vi "testCQTDDSlabview.vi"() -> ()   [LabVIEW 2009, in "run.lvlib"]
uses:
  run.lvlib
  Channels/DDSOutput/Generic/DDSOutput.lvclass
panel:
  in  "Phase 2":dbl[](array[numeric])=[0.0, 0.0, 0.0]
  in  "Amp 2":dbl[](array[numeric])=[1.0, 1.0, 0.0]
  in  "freq 2":dbl[](array[numeric])=[100.0, 90.0, 100.0]
  in  "Phase":dbl[](array[numeric])=[0.0, 0.0, 0.0]
  in  "Amp":dbl[](array[numeric])=[1.0, 1.0, 0.0]
  in  "freq":dbl[](array[numeric])=[100.0, 90.0, 100.0]
  in  "Times":dbl[](array[numeric])=[0.0, 1.0, 2.0]
  in  "stop":bool
  in  "physicalChannels":string[](array[string])=["CQTDDS0_rf_00", "CQTDDS0_rf_01"]
  in  "data":T1(array[cluster])=[{"Frequency(MHz)"=10.0, "Amplitude"=1.0, "Phase"=0.0, "OutputForm"=enum."Sine"}, {"Frequency(MHz)"=10.0, "Amplitude"=1.0, "Phase"=180.0, "OutputForm"=enum."Sine"}]
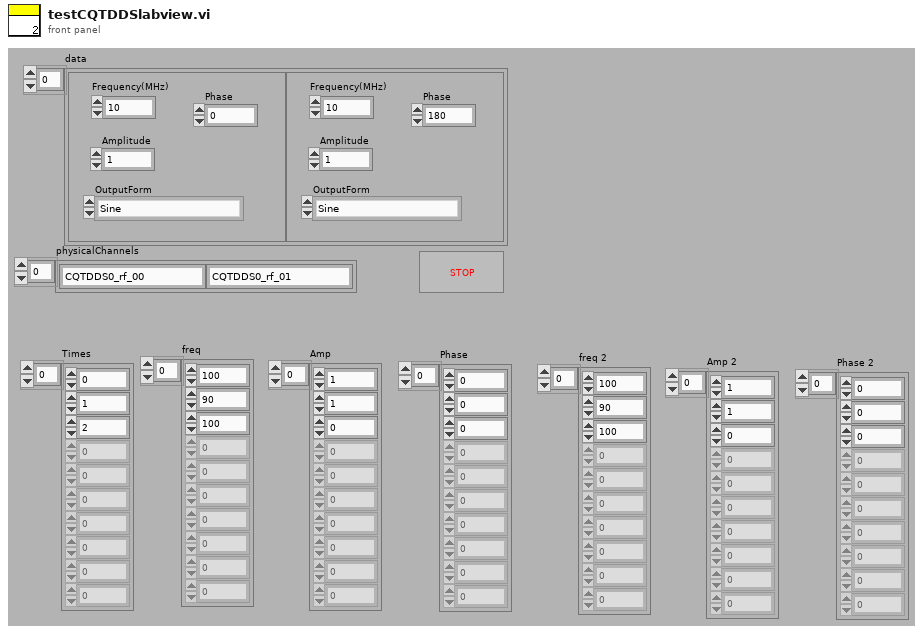
[diagram p1: front panel]
types:
  T1 = cluster{"Frequency(MHz)":dbl, "Amplitude":dbl, "Phase":dbl, "OutputForm":enum16{"Sine", "Square", "Triangle", "Arbitrary"}}[]
  T2 = cluster{"OutputForm":enum16{"Sine", "Square", "Triangle", "Arbitrary"}[], "OutputFunction":enum16{"Frequency", "Ramp", "Sequence"}[], "physicalChannels":string}
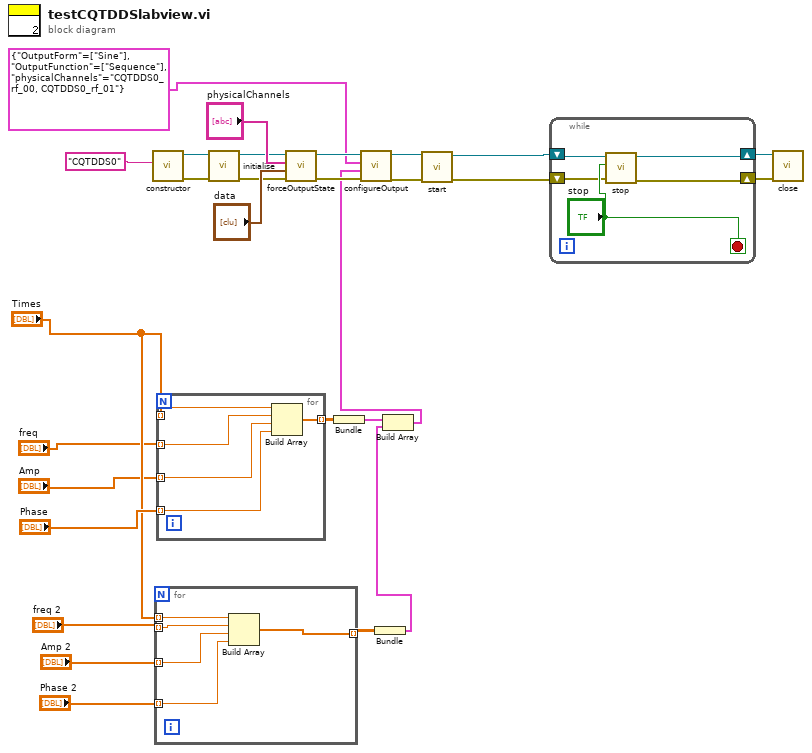
[diagram p0: block diagram]
diagram:
  n1 = call "constructor.vi"("device"="CQTDDS0") -> ("error out"=w22:errorcluster, "DDSOutput out"=w23:refnum<class "DDSOutput.lvclass">)  [unwired: 9 in]
  n2 = for {
    tunnel: "Times" -> [w33] mode=indexing
    tunnel: "freq 2" -> [w32] mode=indexing
    tunnel: "Amp 2" -> [w31] mode=indexing
    tunnel: "Phase 2" -> [w30] mode=indexing
    tunnel: [w29] -> w6 mode=indexing
    n3 = Build Array(w33, w32, w31, w30) -> (w29:dbl[])
  }
  n4 = for {
    tunnel: "Times" -> [w38] mode=indexing
    tunnel: "freq" -> [w37] mode=indexing
    tunnel: "Amp" -> [w35] mode=indexing
    tunnel: "Phase" -> [w34] mode=indexing
    tunnel: [w36] -> w19 mode=indexing
    n5 = Build Array(w38, w37, w35, w34) -> (w36:dbl[])
  }
  n6 = call-dynamic "initialise.vi"("error in (no error)"=w22, "DDSOutput in"=w23) -> ("error out"=w20:errorcluster, "DDSOutput out"=w21:refnum<class "DDSOutput.lvclass">)  [unwired: 8 in]
  n7 = call-dynamic "forceOutputState.vi"("error in (no error)"=w20, "data"="data", "physicalChannels"="physicalChannels", "DDSOutput in"=w21) -> ("error out"=w15:errorcluster, "DDSOutput out"=w16:refnum<class "DDSOutput.lvclass">)  [unwired: 6 in]
  n8 = Bundle(w19) -> (w18:cluster{dbl[][]})  [unwired: 1 in]
  n9 = Bundle(w6) -> (w5:cluster{dbl[][]})  [unwired: 1 in]
  n10 = Build Array(w18, w5) -> (w13:cluster{dbl[][]}[])
  n11 = call-dynamic "configureOutput.vi"("error in (no error)"=w15, "Data"=w13, "Config"=T2 {"OutputForm"=[enum."Sine"], "OutputFunction"=[enum."Sequence"], "physicalChannels"="CQTDDS0_rf_00, CQTDDS0_rf_01"}, "DDSOutput in"=w16) -> ("error out"=w11:errorcluster, "DDSOutput out"=w12:refnum<class "DDSOutput.lvclass">)  [unwired: 6 in]
  n12 = call-dynamic "start.vi"("error in (no error)"=w11, "DDSOutput in"=w12) -> ("error out"=w9:errorcluster, "DDSOutput out"=w10:refnum<class "DDSOutput.lvclass">)  [unwired: 8 in]
  n13 = while {
    shift-right: [w42] -> w25
    shift-left: w10 -> [w43]
    shift-right: [w39] -> w24
    shift-left: w9 -> [w40]
    stop <- "stop" stop-if-true
    n14 = call-dynamic "stop.vi"("error in (no error)"=w40, "stop?"="stop", "DDSOutput in"=w43) -> ("error out"=w39:errorcluster, "DDSOutput out"=w42:refnum<class "DDSOutput.lvclass">)  [unwired: 6 in, 1 out]
  }
  n15 = call-dynamic "close.vi"("error in (no error)"=w24, "DDSOutput in"=w25) -> ()  [unwired: 9 in, 1 out]
